vi "AssertAllItems.vi"(0 "VI Reference In":refnum<vi>, 1 "Test Label":string, 2 "delimiter (>>)":string=">>", 3 "Assert Only? (F)":bool, 5 "Control Path":string, 7 "Item Names":string[][](array[string]), 9 "Ignore Order? (F)":bool, 11 "Error In":errorcluster, 12 "Assert Interval(10 ms)":u32=10, 13 "Timeout(5 sec)":dbl=5.0) -> (4 "VI Reference Out":refnum<vi>, 6 "Asserted Value":string[][](array[string]), 15 "Error Out":errorcluster)   [LabVIEW 2016, in "Drona.lvlib" / "AssertControlValue.lvlib" / "AssertMCListbox.lvlib"]
doc: "Asserts if all the items present in the multi-column listbox control are equal.\n\nThe input control name is given as a string, incase of the path, use delimiters in between the path.\nThis VI gets the control value until the value is equal to the input value."
uses:
  AssertMCListbox.lvlib
  Get/GetControlRef/GetControlRefByPath.vi
  <vilib>/addons/_JKI Toolkits/Caraya/classes/Assert/Assert Equal Value_Variant.vi
  <vilib>/Utility/error.llb/Error Cluster From Error Code.vi
  <vilib>/ErrorRing/Error Ring.xnode
  <vilib>/addons/_JKI Toolkits/Caraya/classes/Assert/Assert.lvclass
  Get/GetControlRef/GetControlRef.lvlib
  <vilib>/SLL Toolkit/SLL String/SLL String.lvlib
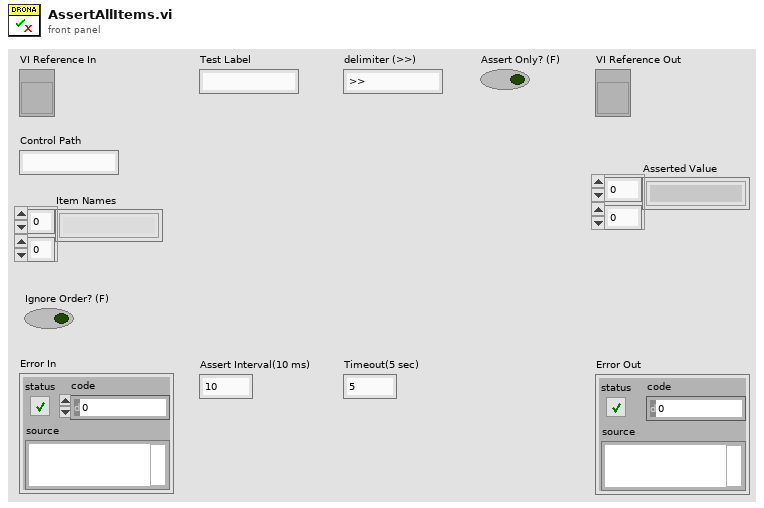
[diagram p1: front panel]
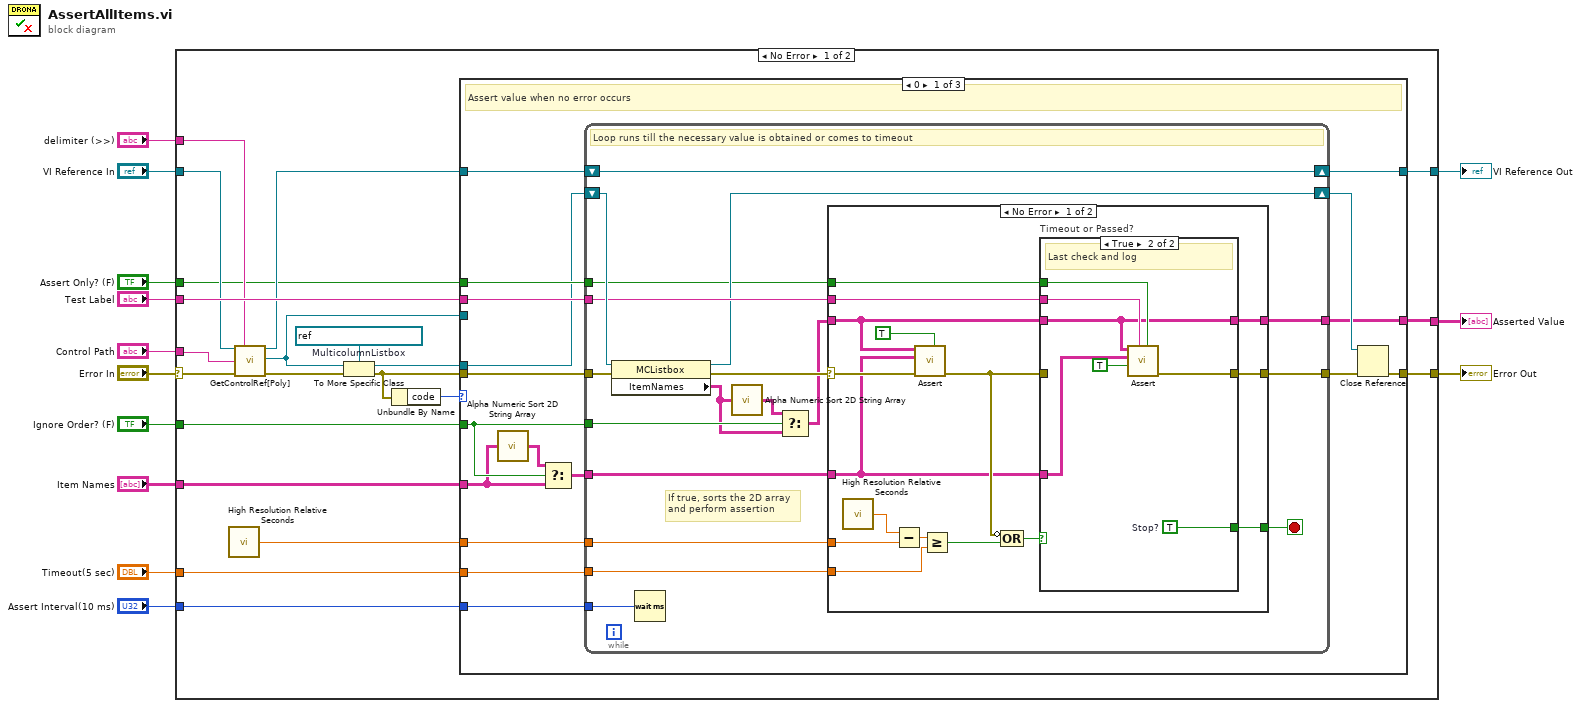
[diagram p0: block diagram]
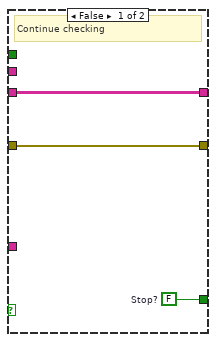
[diagram p2: hidden frame]
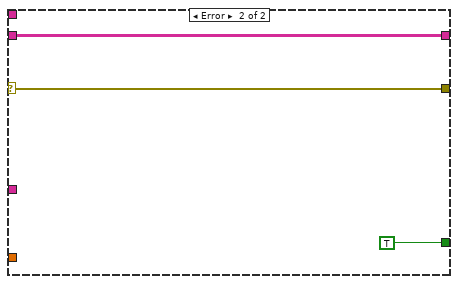
[diagram p3: hidden frame]
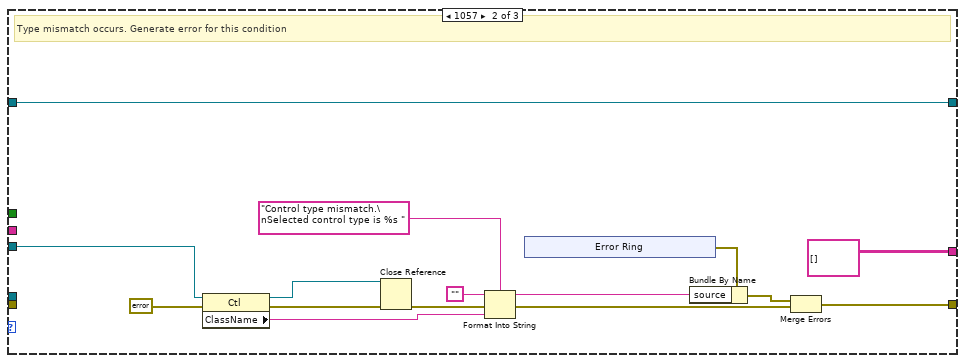
[diagram p4: hidden frame]
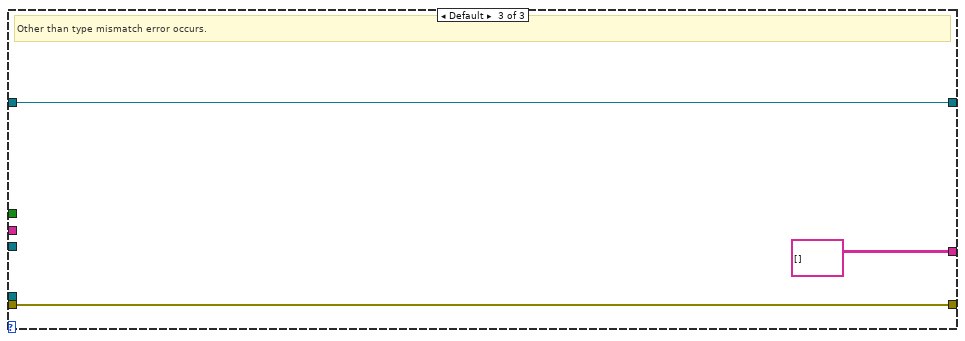
[diagram p5: hidden frame]
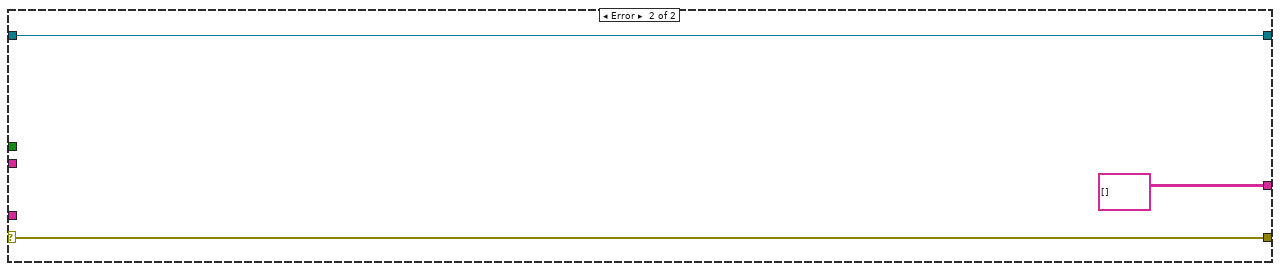
[diagram p6: hidden frame]
diagram:
  n1 = case shown="No Error" "Error In" {
    selector: "Error In" -> [w30 w124]
    tunnel: "Timeout(5 sec)" -> [w34 _]
    tunnel: [w33 w123] -> w12
    tunnel: [w24 w124] -> w11
    tunnel: "Assert Interval(10 ms)" -> [w32 _]
    tunnel: "Test Label" -> [w31 _]
    tunnel: "VI Reference In" -> [w29 w123]
    tunnel: "Control Path" -> [w28 _]
    tunnel: "delimiter (>>)" -> [w23 _]
    tunnel: "Assert Only? (F)" -> [w22 _]
    tunnel: [w21 string[][] [] ("Item Names")] -> w2
    tunnel: "Item Names" -> [w18 _]
    tunnel: "Ignore Order? (F)" -> [w14 _]
    frame No Error {
      w20 = refnum<vi> refnum  # MulticolumnListbox
      n2 = call <vilib>:"High Resolution Relative Seconds.vi"() -> ("relative seconds"=w27:dbl)
      n3 = call-poly "GetControlRef[Poly].vi"("VI Reference In"=w29, "delimiter (>>)"=w23, "Control Path"=w28, "error In"=w30) -> ("VI Reference Out"=w25:refnum<vi>, "Ctl Refnum"=w15:refnum<vi>, "error out"=w26:errorcluster)  [unwired: 9 in]
      n4 = To More Specific Class(target class=w20, reference=w15, error in=w26) -> (specific class reference=w19:refnum<vi>, error out=w17:errorcluster)
      n5 = Unbundle By Name(w17) -> ("code"=w16:i32)
      n6 = case shown="0" w16 {
        tunnel: w34 -> [w51 _ _]
        tunnel: [w50 w112 w121] -> w33
        tunnel: w32 -> [w48 _ _]
        tunnel: w31 -> [w47 _ _]
        tunnel: w27 -> [w46 _ _]
        tunnel: w25 -> [w45 w112 w121]
        tunnel: [w44 w100 w120] -> w24
        tunnel: w22 -> [w42 _ _]
        tunnel: [w41 string[][] [] ("Item Names") string[][] [] ("Item Names")] -> w21
        tunnel: w17 -> [w40 _ w120]
        tunnel: w19 -> [w39 _ _]
        tunnel: w18 -> [w35 _ _]
        tunnel: w15 -> [_ w99 _]
        tunnel: w14 -> [w37 _ _]
        frame 0 {
          # "Assert value when no error occurs"
          n7 = call <vilib>:"Alpha Numeric Sort 2D String Array.vi"("2D String[]"=w35) -> ("Sorted 2D String[]"=w36:string[][])  [unwired: 3 in, 1 out]
          n8 = Select(t=w36, s=w37, f=w35) -> (s? t:f=w38:string[][])
          n9 = while {
            tunnel: w51 -> [w68]
            tunnel: w46 -> [w69]
            tunnel: w40 -> [w63]
            tunnel: [w66] -> w49
            tunnel: w48 -> [w64]
            tunnel: w47 -> [w60]
            shift-right: [w61] -> w50
            shift-left: w45 -> [w61]
            shift-right: [w59] -> w43
            shift-left: w39 -> [w62]
            tunnel: w42 -> [w58]
            tunnel: [w57] -> w41
            tunnel: w38 -> [w56]
            tunnel: w37 -> [w55]
            stop <- w67 stop-if-true
            # "If true, sorts the 2D array \nand perform assertion"
            # "Loop runs till the necessary value is obtained or comes to timeout"
            n10 = property on="Property Node" class="MCListbox"(reference=w62, error in=w63) -> (reference out=w59:refnum<vi>, error out=w65:errorcluster, "ItemNames"=w53:string[][])
            n11 = Wait (ms)(milliseconds to wait=w64) -> ()  [unwired: 1 out]
            n12 = call <vilib>:"Alpha Numeric Sort 2D String Array.vi"("2D String[]"=w53) -> ("Sorted 2D String[]"=w52:string[][])  [unwired: 3 in, 1 out]
            n13 = Select(t=w52, s=w55, f=w53) -> (s? t:f=w54:string[][])
            n14 = case shown="No Error" w65 {
              selector: w65 -> [w81 w98]
              tunnel: w69 -> [w85 _]
              tunnel: w68 -> [w82 _]
              tunnel: [w73 TRUE] -> w67
              tunnel: [w74 w98] -> w66
              tunnel: w54 -> [w75 w96]
              tunnel: w60 -> [w80 _]
              tunnel: w58 -> [w72 _]
              tunnel: [w71 w96] -> w57
              tunnel: w56 -> [w70 _]
              frame No Error {
                n15 = call <vilib>:"High Resolution Relative Seconds.vi"() -> ("relative seconds"=w84:dbl)
                n16 = Subtract(x=w84, y=w85) -> (x-y=w83:dbl)
                n17 = call-poly <vilib>:"Assert.vi"("Assert Only? (F)"=TRUE, "error in (no error)"=w81, "Y"=w70, "X"=w75) -> ("error out"=w78:errorcluster)  [unwired: 6 in, 1 out]
                n18 = Greater Or Equal?(x=w83, y=w82) -> (x >= y?=w79:bool)
                n19 = Compound Arithmetic op=OR(invert w78, w79) -> (w77:bool)
                n20 = case "Timeout or Passed?" shown="True" w77 {
                  tunnel: w78 -> [w88 _]
                  tunnel: w70 -> [_ w94]
                  tunnel: w75 -> [w86 w89]
                  tunnel: w80 -> [_ w95]
                  tunnel: [w88 w93] -> w74
                  tunnel: [w87 w92] -> w73
                  tunnel: w72 -> [_ w90]
                  tunnel: [w86 w89] -> w71
                  frame False {
                    w87 = FALSE  # Stop?
                    # "Continue checking"
                  }
                  frame True {
                    w92 = TRUE  # Stop?
                    # "Last check and log"
                    n21 = call-poly <vilib>:"Assert.vi"("Assert Only? (F)"=w90, "Label"=w95, "Register with caller test (F)"=TRUE, "Y"=w94, "X"=w89) -> ("error out"=w93:errorcluster)  [unwired: 5 in, 1 out]
                  }
                }
              }
              frame Error {
              }
            }
          }
          n22 = Close Reference(reference=w43, error in (no error)=w49) -> (error out=w44:errorcluster)
        }
        frame 1057 {
          # "Type mismatch occurs. Generate error for this condition"
          n23 = property class="Ctl"(reference=w99, error in=errorcluster {"status"=FALSE, "code"=0, "source"=""} ("error out")) -> (reference out=w101:refnum<vi>, error out=w111:errorcluster, "ClassName"=w108:string)
          n24 = Close Reference(reference=w101, error in (no error)=w111) -> (error out=w102:errorcluster)
          n25 = Format Into String(format string="Control type mismatch.\nSelected control type is %s ", initial string="", error in=w102, w108) -> (resulting string=w105:string, error out=w103:errorcluster)
          n26 = xnode "Error Ring"() -> ("error out"=w106:errorcluster)
          n27 = Bundle By Name(cluster=w106, "source"=w105) -> (w104:errorcluster)
          n28 = Merge Errors(w104, w103) -> (w100:errorcluster)
        }
        frame Default {
          # "Other than type mismatch error occurs."
        }
      }
    }
    frame Error {
    }
  }
  "Error Out" <- w11
  "VI Reference Out" <- w12
  "Asserted Value" <- w2
